vi "Upshift MLE Baseline.vi"(7 "NL Fit Method":T6, 8 "MLE Fit Options":T1, 9 "All Parameter Constraints in":T3, 10 "Data in":dbl[](array[numeric]), 11 "Guess parameters in":dbl[](array[numeric])) -> (0 "MLE_Baseline_Offset out":dbl=1.0 format="%#_13g", 1 "All Parameter Constraints out":T3, 2 "Data out":dbl[](array[numeric]), 3 "Guess parameters out":dbl[](array[numeric]))   [LabVIEW 2021, in "Fits.lvlib"]
uses:
  Fits.lvlib
  Nonlinear Fit Method.ctl
  Decay Fit Parameter Constraints Arrays.ctl
  Decay Fit Parameters In List.ctl
  Decay Convolution/Decay Model.ctl
  MLE Fit Options.ctl
  MLE Baseline Offset Type.ctl
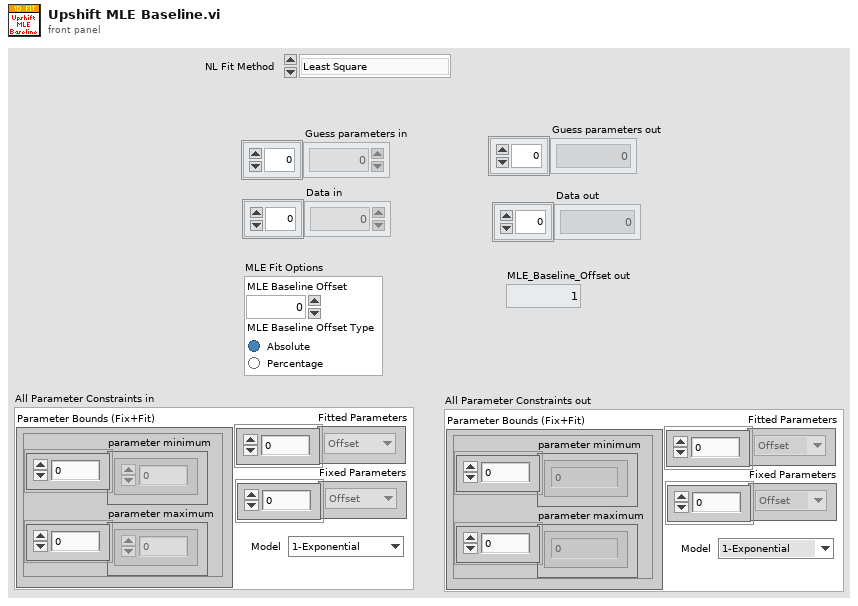
[diagram p1: front panel]
types:
  T1 = typedef "Fits.lvlib/MLE Fit Options.ctl" = cluster{"MLE Baseline Offset":dbl, "MLE Baseline Offset Type":T2}
  T2 = typedef "Fits.lvlib/MLE Baseline Offset Type.ctl" = enum32{"Absolute", "Percentage"}
  T3 = typedef "Fits.lvlib/Decay Fit Parameter Constraints Arrays.ctl" = cluster{"Parameter Bounds (Fix+Fit)":cluster{"parameter minimum":dbl[], "parameter maximum":dbl[]}, "Fitted Parameters":T4[], "Fixed Parameters":T4[], "Fit Model":T5}
  T4 = typedef "Fits.lvlib/Decay Fit Parameters In List.ctl" = enum16{"Offset", "Baseline", "A_1", "tau_1", "A_2", "tau_2"}
  T5 = typedef "Fits.lvlib/Decay Model.ctl" = enum16{"1-Exponential", "2-Exponentials"}
  T6 = typedef "Fits.lvlib/Nonlinear Fit Method.ctl" = enum16{"Least Square", "Least Absolute Residual", "Bisquare", "MLE"}
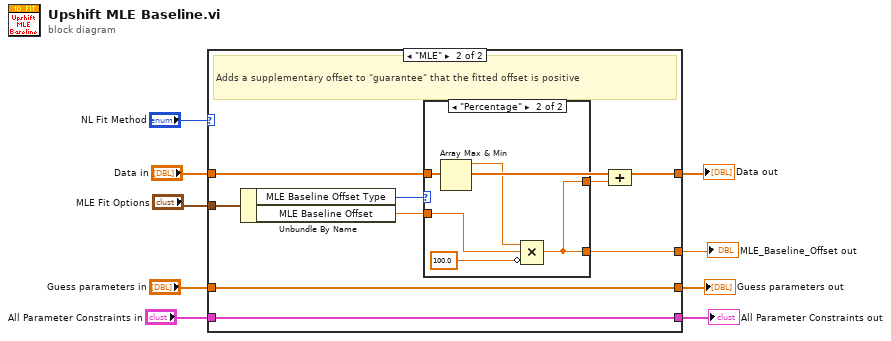
[diagram p0: block diagram]
diagram:
  n1 = case shown="\"MLE\"" "NL Fit Method" {
    tunnel: "Data in" -> [w12 w16]
    tunnel: [w12 w21] -> w7
    tunnel: "Guess parameters in" -> [w11 w20]
    tunnel: [w11 w20] -> w5
    tunnel: "All Parameter Constraints in" -> [w10 w19]
    tunnel: [w10 w19] -> w3
    tunnel: [_ w17] -> w2
    tunnel: "MLE Fit Options" -> [_ w15]
    frame "Least Square", Default {
    }
    frame "MLE" {
      # "Adds a supplementary offset to \"guarantee\" that the fitted offset is positive"
      n2 = Unbundle By Name(w15) -> ("MLE Baseline Offset Type"=w14:T2, "MLE Baseline Offset"=w13:dbl)
      n3 = case shown="\"Percentage\"" w14 {
        tunnel: [w22 w26] -> w18
        tunnel: [w22 w26] -> w17
        tunnel: w16 -> [_ w25]
        tunnel: w13 -> [w22 w23]
        frame "Absolute", Default {
        }
        frame "Percentage" {
          n4 = Array Max & Min(array=w25) -> (max value=w24:dbl)  [unwired: 3 out]
          n5 = Compound Arithmetic op=MULTIPLY(w24, w23, invert 100.0 ("value")) -> (w26:dbl)
        }
      }
      n6 = Compound Arithmetic op=ADD(w16, w18) -> (w21:dbl[])
    }
  }
  "Guess parameters out" <- w5
  "Data out" <- w7
  "All Parameter Constraints out" <- w3
  "MLE_Baseline_Offset out" <- w2
